vi "Compute Weight Array v2.vi"(8 "Error In":errorcluster, 9 "Weighted Fit":bool, 10 "Control Data Array":dbl[](array[numeric]), 11 "Data Array":dbl[](array[numeric])) -> (0 "Error Out":errorcluster, 3 "Weight Array":dbl[](array[numeric]))   [LabVIEW 2019]
doc: "If provided, the control array should have the same dimension as the data array and be in [0, 1]"
panel:
  # "<--------- between 0 and 1"
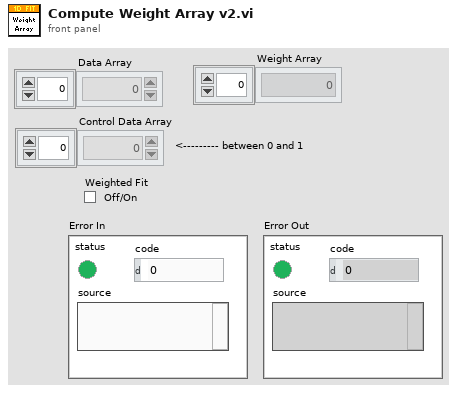
[diagram p1: front panel]
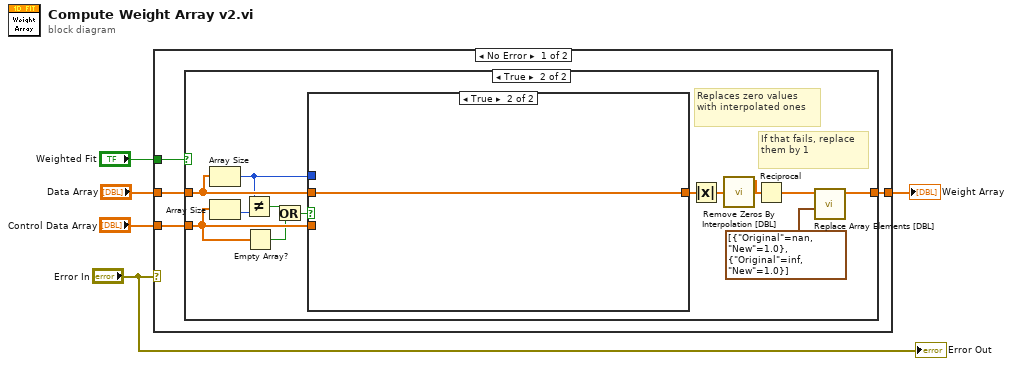
[diagram p0: block diagram]
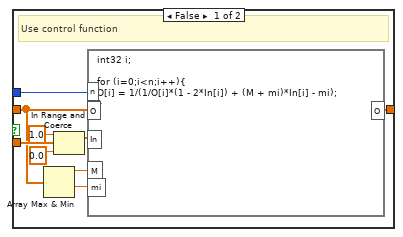
[diagram p3: hidden frame]
diagram:
  n1 = case shown="No Error" "Error In" {
    tunnel: [w9 _] -> w5
    tunnel: "Data Array" -> [w7 _]
    tunnel: "Weighted Fit" -> [w8 _]
    tunnel: "Control Data Array" -> [w6 _]
    frame No Error {
      n2 = case shown="True" w8 {
        tunnel: [_ w22] -> w9
        tunnel: w7 -> [_ w18]
        tunnel: w6 -> [_ w17]
        frame False {
        }
        frame True {
          # "If that fails, replace them by 1"
          # "Replaces zero values with interpolated ones"
          n3 = Array Size(array=w18) -> (size(s)=w12:i32)
          n4 = Array Size(array=w17) -> (size(s)=w16:i32)
          n5 = Not Equal?(x=w12, y=w16) -> (x != y?=w15:bool)
          n6 = Empty Array?(array=w17) -> (empty?=w14:bool)
          n7 = Or(x=w15, y=w14) -> (x .or. y?=w13:bool)
          n8 = case shown="True" w13 {
            tunnel: w18 -> [w25 w32]
            tunnel: [w26 w32] -> w19
            tunnel: w17 -> [w31 _]
            tunnel: w12 -> [w27 _]
            frame False {
              # "Use control function"
              n9 = Array Max & Min(array=w25) -> (max value=w24:dbl, min value=w23:dbl)  [unwired: 2 out]
              n10 = In Range and Coerce(upper limit=1.0, x=w31, lower limit=0.0 ("upper limit")) -> (coerced(x)=w28:dbl[])  [unwired: 1 out]
              n11 = formula code="int32 i;\n\nfor (i=0;i<n;i++){\nO[i] = 1/(1/O[i]*(1 - 2*In[i]) + (M + mi)*In[i] - mi);\n}"("O"=w25, "In"=w28, "n"=w27, "M"=w24, "mi"=w23) -> ("O"=w26:dbl[])
            }
            frame True {
            }
          }
          n12 = Absolute Value(x=w19) -> (abs(x)=w20:dbl[])
          n13 = call "Remove Zeros By Interpolation [DBL].vi"("Array in"=w20) -> ("Array out"=w11:dbl[])  [unwired: 9 in, 1 out]
          n14 = Reciprocal(x=w11) -> (1/x=w21:dbl[])
          n15 = call "Replace Array Elements [DBL].vi"("Array of Replacement Pairs"=cluster{"Original":dbl, "New":dbl}[] [{"Original"=nan, "New"=1.0}, {"Original"=inf, "New"=1.0}], "Array"=w21) -> ("Array with Replacements"=w22:dbl[])  [unwired: 9 in]
        }
      }
    }
    frame Error {
    }
  }
  "Weight Array" <- w5
  "Error Out" <- "Error In"
